vi "Enqueue Array of Events.vi"(8 "error in (no error)":errorcluster, 10 "Events":T1[](array[typedef]), 11 "Queue in":refnum<queue>) -> (0 "error out":errorcluster)   [LabVIEW 2017, in "Test Bench.lvlib"]
uses:
  Test Bench.lvlib
  Action States.ctl
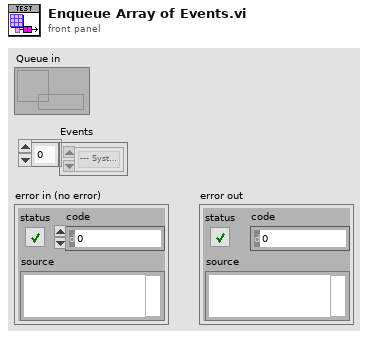
[diagram p1: front panel]
types:
  T1 = typedef "Test Bench.lvlib/Action States.ctl" = enum16{"--- System ---", "Reset", "Exit", "--- File ---", "Load Table from File", "--- DIO ---", "Update DIO Registers", "Read DI States", "--- AO ---", "Select Target AO Channel", "Update Idle Voltage", "Update AO Generation Method", "Update Update Rate", "Update Waveform Increment", "Update Waveform Table"}
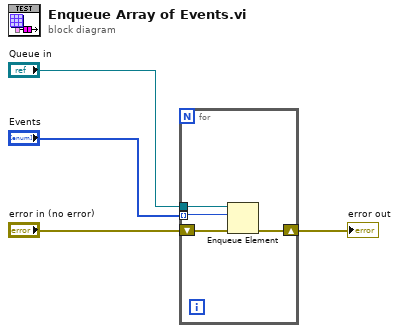
[diagram p0: block diagram]
diagram:
  n1 = for {
    tunnel: "Queue in" -> [w7]
    shift-right: [w8] -> w4
    shift-left: "error in (no error)" -> [w6]
    tunnel: "Events" -> [w5] mode=indexing
    n2 = Enqueue Element(queue=w7, element=w5, error in (no error)=w6) -> (error out=w8:errorcluster)  [unwired: 1 in, 2 out]
  }
  "error out" <- w4
